vi "Open output.vi"(8 "error in (no error)":errorcluster, 10 "Pipe buffer size":u32=30 min=4, 11 "STD IN/OUT":u32(ring)=4294967284 items=["STD_OUTPUT_HANDLE"=4294967285, "STD_ERROR_HANDLE"=4294967284]) -> (0 "error out":errorcluster, 1 "Write handle":u64, 2 "Read handle":u64, 3 "Original handle":u64)   [LabVIEW 2012, in "LightPipes.lvlib"]
uses:
  LightPipes.lvlib
  kernel32.dll
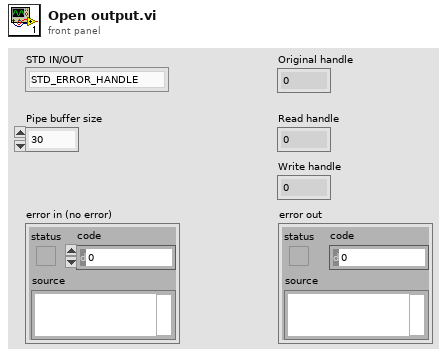
[diagram p1: front panel]
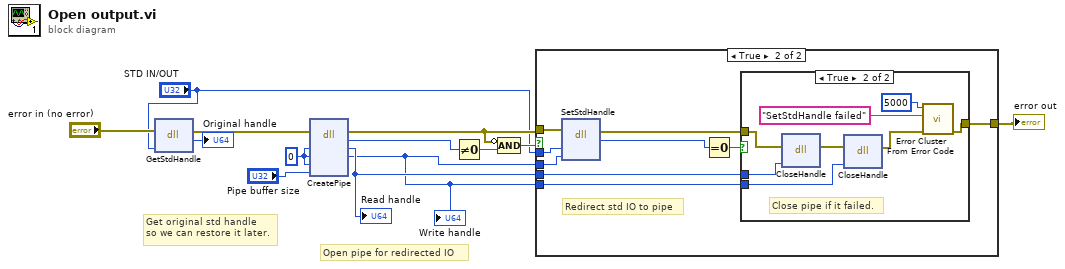
[diagram p0: block diagram]
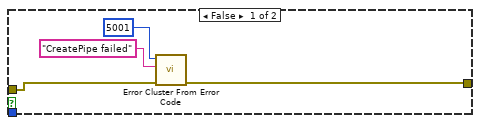
[diagram p2: hidden frame]
diagram:
  w12 = u64 0 ("hReadPipe")
  # "Open pipe for redirected IO"
  # "Get original std handle\nso we can restore it later."
  n1 = dll-call lib="kernel32.dll" fn="GetStdHandle"(error in="error in (no error)", "nStdHandle"="STD IN/OUT") -> (error out=w7:errorcluster, "HANDLE"=→"Original handle":u64)  [unwired: 3 in, 1 out]
  n2 = dll-call lib="kernel32.dll" fn="CreatePipe"(error in=w7, "hReadPipe"=w12, "hWritePipe"=w12, "lpPipeAttributes"=w12, "nSize"="Pipe buffer size") -> (error out=w10:errorcluster, "BOOL"=w9:i32, "hReadPipe"=w3:u64, "hWritePipe"=w2:u64)  [unwired: 4 in, 1 out]
  "Read handle" <- w3
  "Write handle" <- w2
  n3 = Not Equal To 0?(x=w9) -> (x != 0?=w11:bool)
  n4 = Compound Arithmetic op=AND(invert w10, w11) -> (w8:bool)
  n5 = case shown="True" w8 {
    tunnel: w2 -> [_ w26]
    tunnel: w10 -> [w15 w25]
    tunnel: "STD IN/OUT" -> [_ w24]
    tunnel: [w14 w18] -> w1
    tunnel: w3 -> [_ w20]
    tunnel: w2 -> [_ w19]
    frame False {
      n6 = call <vilib>:"Error Cluster From Error Code.vi"("error in (no error)"=w15, "error message (\"\")"="CreatePipe failed" ("error message (\"\")"), "error code (0)"=5001) -> ("error out"=w14:errorcluster)  [unwired: 6 in]
    }
    frame True {
      # "Redirect std IO to pipe"
      n7 = dll-call lib="kernel32.dll" fn="SetStdHandle"(error in=w25, "nStdHandle"=w24, "hHandle"=w26) -> (error out=w21:errorcluster, "BOOL"=w23:i32)  [unwired: 4 in, 1 out]
      n8 = Equal To 0?(x=w23) -> (x = 0?=w22:bool)
      n9 = case shown="True" w22 {
        tunnel: w21 -> [w27 w33]
        tunnel: w20 -> [_ w30]
        tunnel: w19 -> [_ w29]
        tunnel: [w27 w28] -> w18
        frame False {
        }
        frame True {
          # "Close pipe if it failed."
          n10 = dll-call lib="kernel32.dll" fn="CloseHandle"(error in=w33, "hObject"=w30) -> (error out=w32:errorcluster)  [unwired: 4 in, 1 out]
          n11 = dll-call lib="kernel32.dll" fn="CloseHandle"(error in=w32, "hObject"=w29) -> (error out=w31:errorcluster)  [unwired: 4 in, 1 out]
          n12 = call <vilib>:"Error Cluster From Error Code.vi"("error in (no error)"=w31, "error message (\"\")"="SetStdHandle failed" ("error message (\"\")"), "error code (0)"=5000) -> ("error out"=w28:errorcluster)  [unwired: 6 in]
        }
      }
    }
  }
  "error out" <- w1
